vi "initialize.vi"(7 "Ref Point":cluster{"X Ref":dbl, "Y Ref":dbl} {"Y Ref" min=-8.0 max=8.0; "X Ref" min=-8.0 max=8.0}, 8 "Data Savefile Path":path=path "/home/lvuser/logs.bin", 9 "path refs":path=path "/home/lvuser/home/lvuser/Meebed/DDcontroller.bin", 10 "Cluster":T1={"Frequency Divider"=5, "Periods"=8, "Order"=5, "Reference "=0, "Amplitude"=0.5} {"Amplitude" min=0.0; "Reference" items=["Change X", "Change Y"]; "Order" min=1 step=1; "Periods" min=1 step=1; "Frequency Divider" min=1 step=1}, 11 "mode":T2) -> (3 "Qube":refnum<class "System.lvclass">)   [LabVIEW 2021, in "System.lvclass"]
uses:
  System.lvclass
  mode.ctl
  System.lvclass/System.ctl
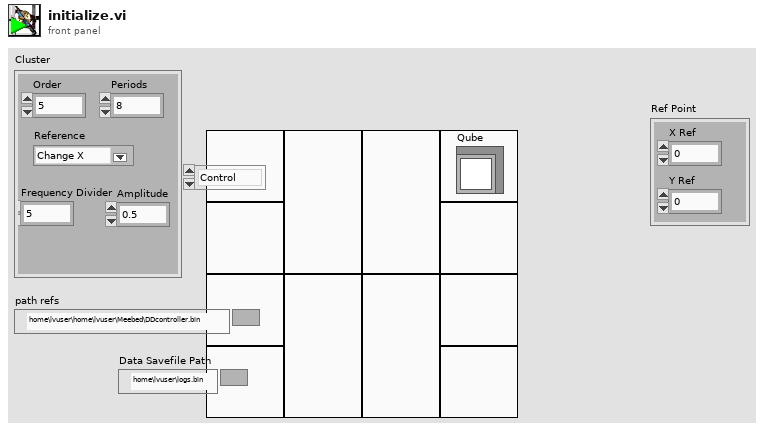
[diagram p1: front panel]
types:
  T1 = cluster{"Frequency Divider":u32, "Periods":u32, "Order":u32, "Reference ":u16, "Amplitude":dbl}
  T2 = typedef "System.lvclass/mode.ctl" = enum16{"Control", "Identify"}
  T3 = enum16{"open", "replace", "create", "open or create", "replace or create", "replace or create with confirmation"}
  T4 = enum16{"big-endian, network order", "native, host order", "little-endian"}
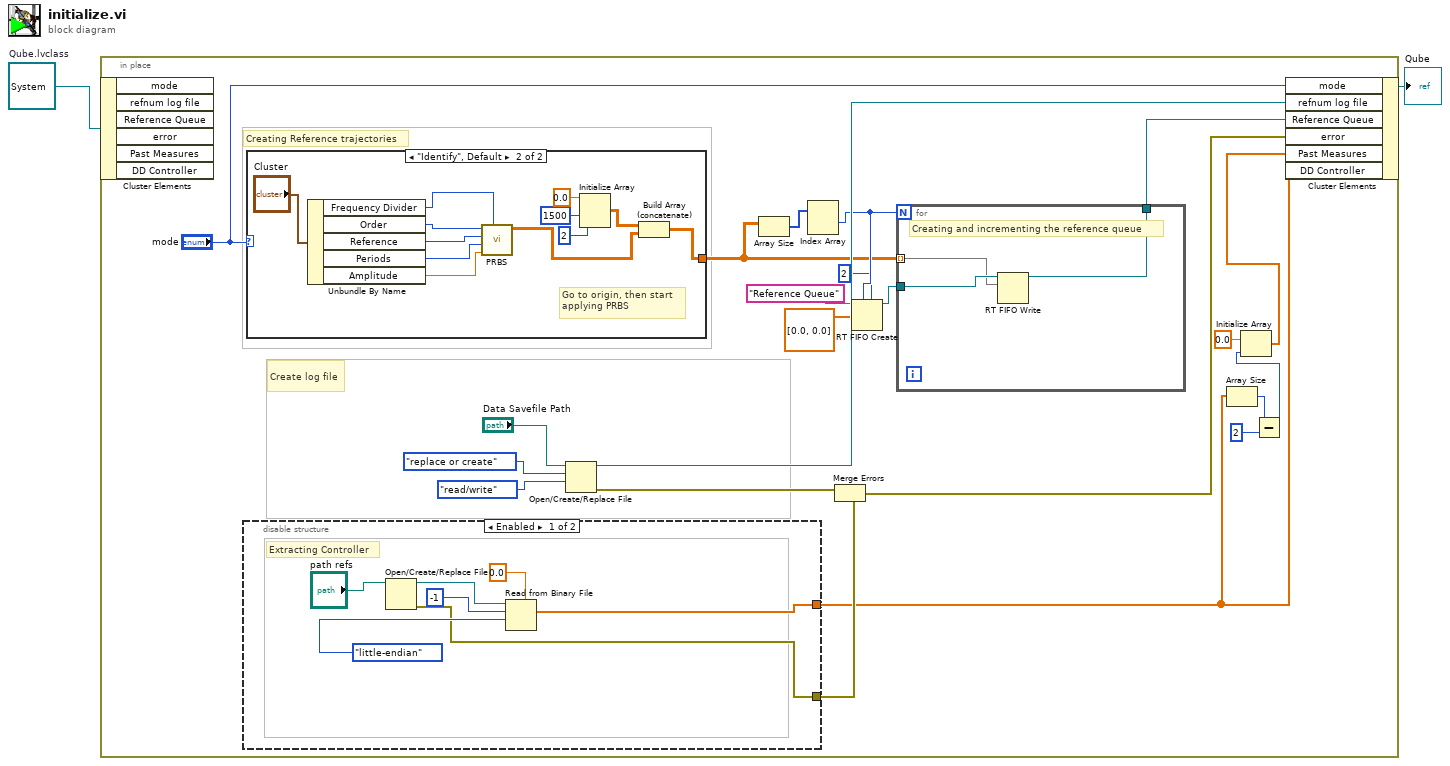
[diagram p0: block diagram]
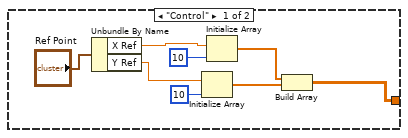
[diagram p3: hidden frame]
diagram:
  w1 = refnum<class "System.lvclass"> refnum  # Qube.lvclass
  n1 = in-place {
    # "Creating Reference trajectories"
    # "Create log file"
    n2 = in-place-cluster #1(w1) -> ()  [unwired: 6 out]
    n3 = disable-structure shown="Enabled" {
      disable-tunnel: [w30 _] -> w24
      disable-tunnel: [w28 _] -> w8
      frame Enabled {
        # "Extracting Controller"
        n4 = Open/Create/Replace File(file path (use dialog)="path refs") -> (refnum out=w34:refnum<file>, error out=w30:errorcluster)  [unwired: 5 in, 1 out]
        n5 = Read from Binary File(5:0.0, 9:T4."little-endian" ("byte order (0:big-endian, network order)"), 10:-1 ("count (1)"), 11:w34) -> (2:w28:dbl[])  [unwired: 2 in, 3 out]
      }
      frame Disabled {
      }
    }
    n6 = case shown="\"Identify\", Default" "mode" {
      tunnel: [w35 w49] -> w11
      frame "Control" {
        n7 = Unbundle By Name("Ref Point") -> ("X Ref"=w39:dbl, "Y Ref"=w38:dbl)
        n8 = Initialize Array(w38, 10 ("dimension size")) -> (w36:dbl[])
        n9 = Initialize Array(w39, 10 ("dimension size")) -> (w37:dbl[])
        n10 = Build Array(w37, w36) -> (w35:dbl[][])
      }
      frame "Identify", Default {
        # "Go to origin, then start \napplying PRBS"
        n11 = Unbundle By Name("Cluster") -> ("Frequency Divider"=w47:u32, "Order"=w46:u32, "Reference"=w45:u16, "Periods"=w44:u32, "Amplitude"=w43:dbl)
        n12 = call "PRBS.vi"("Frequency Divider"=w47, "Amplitude"=w43, "Periods"=w44, "Reference"=w45, "Order"=w46) -> ("appended array"=w50:dbl[][])  [unwired: 6 in]
        n13 = Initialize Array(0.0 ("element"), 1500 ("dimension size"), 2 ("dimension size")) -> (w51:dbl[][])
        n14 = Build Array (concatenate)(w51, w50) -> (w49:dbl[][])
      }
    }
    n15 = Open/Create/Replace File(file path (use dialog)="Data Savefile Path", operation (0:open)=T3."replace or create", access (0:read/write)=enum16{"read/write", "read-only", "write-only"}."read/write") -> (refnum out=w21:refnum<file>, error out=w23:errorcluster)  [unwired: 3 in, 1 out]
    n16 = Array Size(array=w11) -> (size(s)=w14:i32[])
    n17 = Index Array(array=w14) -> (element #1=w13:i32)  [unwired: 2 in, 1 out]
    n18 = Merge Errors(w23, w24) -> (w22:errorcluster)
    n19 = RT FIFO Create(0:"Reference Queue" ("name (unnamed)"), 1:dbl[] [0.0, 0.0] ("initialized array"), 4:w13, 6:u32 2 ("elements in array (1)")) -> (8:w12:refnum<k33>)  [unwired: 4 in, 2 out]
    n20 = for {
      N: w13 -> [_]
      tunnel: w12 -> [w27]
      tunnel: w11 -> [w26] mode=indexing
      tunnel: [w25] -> w10
      # "Creating and incrementing the reference queue"
      n21 = RT FIFO Write(0:w27, 1:w26) -> (8:w25:refnum<k33>)  [unwired: 3 in, 3 out]
    }
    n22 = Array Size(array=w8) -> (size(s)=w5:i32)
    n23 = Subtract(x=w5, y=2) -> (x-y=w3:i32)
    n24 = Initialize Array(0.0 ("element"), w3) -> (w6:dbl[])
    n25 = in-place-cluster #1("mode"="mode", "refnum log file"=w21, "Reference Queue"=w10, "error"=w22, "Past Measures"=w6, "DD Controller"=w8) -> (→"Qube":refnum<class "System.lvclass">)
  }
